vi "digital-on-delay-test.vi"() -> ()   [LabVIEW 2019]
uses:
  <vilib>/Rock Robotics/WPI/ThirdParty/JAS_Junk/TrajLib/Timer_New.vi
  <vilib>/Utility/semaphor.llb/Obtain Semaphore Reference.vi
  <vilib>/Rock Robotics/WPI/ThirdParty/JAS_Junk/TrajLib/Timer_Reset.vi
  <vilib>/Rock Robotics/WPI/ThirdParty/JAS_Junk/TrajLib/Timer_Start.vi
  <vilib>/Rock Robotics/WPI/ThirdParty/JAS_Junk/TrajLib/Timer_Stop.vi
  <vilib>/Rock Robotics/WPI/ThirdParty/JAS_Junk/TrajLib/Timer_HasPeriodPassedOnce.vi
  <vilib>/Rock Robotics/WPI/ThirdParty/JAS_Junk/TrajLib/Trajectory_Library.lvlib
panel:
  out "Numeric 2":dbl
  out "Ouptut 2":bool
  in  "Delay 2":dbl=3.0
  out "Numeric":dbl
  in  "Delay":dbl=10.0
  out "Ouptut":bool
  in  "Input":bool
  # "ON DELAY TEST"
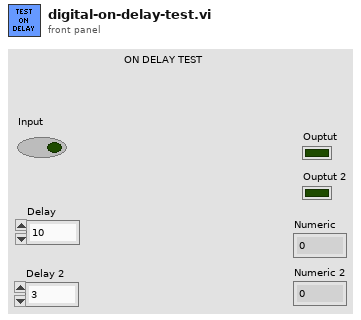
[diagram p1: front panel]
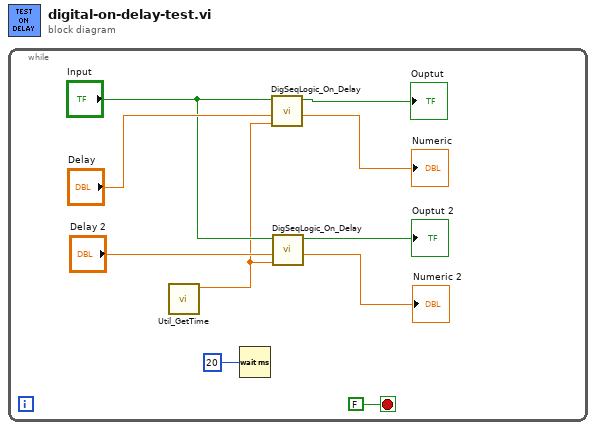
[diagram p0: block diagram]
diagram:
  n1 = while {
    stop <- FALSE stop-if-true
    n2 = call <vilib>:"Util_GetTime.vi"() -> ("FPGA_Time_Seconds"=w1:dbl)  [unwired: 10 in, 1 out]
    n3 = Wait (ms)(milliseconds to wait=u32 20) -> ()  [unwired: 1 out]
    n4 = call <vilib>:"DigSeqLogic_On_Delay.vi"("Time"=w1, "Delay"="Delay", "Input"="Input") -> ("Remain"=→"Numeric":dbl, "Output"=→"Ouptut":bool)  [unwired: 7 in]
    n5 = call <vilib>:"DigSeqLogic_On_Delay.vi"("Time"=w1, "Delay"="Delay 2", "Input"="Input") -> ("Remain"=→"Numeric 2":dbl, "Output"=→"Ouptut 2":bool)  [unwired: 7 in]
  }
